vi "change volume types.vi"(8 "error in (no error)":errorcluster, 10 "change criteria":T2, 11 "manager_daemon in":refnum<class "manager_daemon.lvclass">) -> (0 "error out":errorcluster, 3 "manager_daemon out":refnum<class "manager_daemon.lvclass">)   [LabVIEW 2024, in "manager_daemon.lvclass"]
uses:
  manager_daemon.lvclass
  CV_Shared_Library/volume.type--enum.ctl
  type_defs/msg--cluster.ctl
  type_defs/cmd--enum.ctl
  CV_Shared_Library/CV_Shared_Library.lvlib
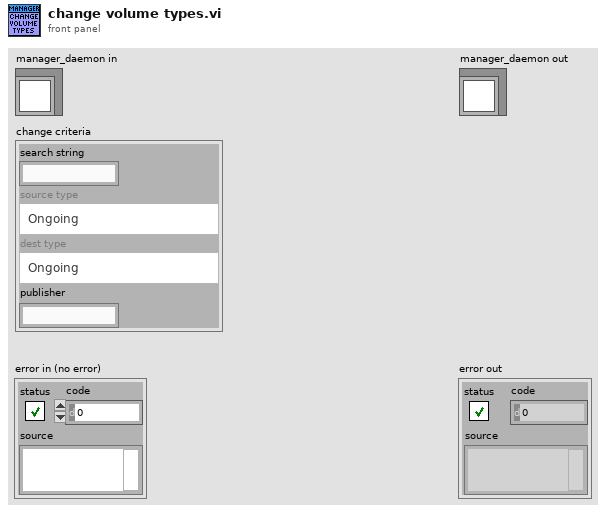
[diagram p1: front panel]
types:
  T1 = typedef "CV_Shared_Library.lvlib/volume.type--enum.ctl" = enum16{"Ongoing", "Limited Series", "Annual", "One Shot", "Reprint/Document", "Digital"}
  T2 = cluster{"search string":string, "source type":T1, "dest type":T1, "publisher":string}
  T3 = typedef "manager_daemon.lvclass/cmd--enum.ctl" = enum16{"init", "run", "load binaries", "save binaries", "updated volume", "get set names", "return vol path by id", "return vol ids by publisher", "display info", "filter release week", "apply filter", "add publisher", "get publishers", "add volume", "add volumes", "add issues", "add issue", "delete volume", "delete issues", "download issues", "scan for reprints", "exit"}
  T4 = typedef "manager_daemon.lvclass/msg--cluster.ctl" = cluster{"cmd":T3, "data":variant}
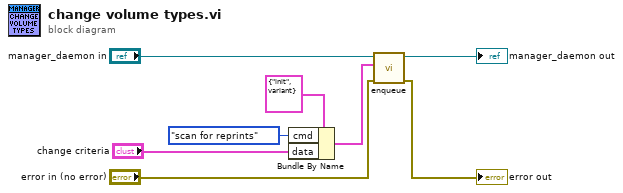
[diagram p0: block diagram]
diagram:
  n1 = Bundle By Name(cluster=T4 {"cmd"=enum."init", "data"=variant} ("msg"), "cmd"=cmd--enum."scan for reprints", "data"="change criteria") -> (w3:T4)
  n2 = call "enqueue.vi"("error in (no error)"="error in (no error)", "msg"=w3, "manager_daemon in"="manager_daemon in") -> ("error out"=→"error out":errorcluster, "manager_daemon out"=→"manager_daemon out":refnum<class "manager_daemon.lvclass">)  [unwired: 7 in]
